vi "prueba.vi"() -> ()   [LabVIEW 2020]
uses:
  <vilib>/userDefined/High Color/IMAQdx.ctl
  <vilib>/vision/driver/NI_Vision_Acquisition_Software.lvlib
panel:
  in  "confirmar":bool
  in  "Session In":T1
  in  "stop":bool
  out "Image":T2(plugin-control)
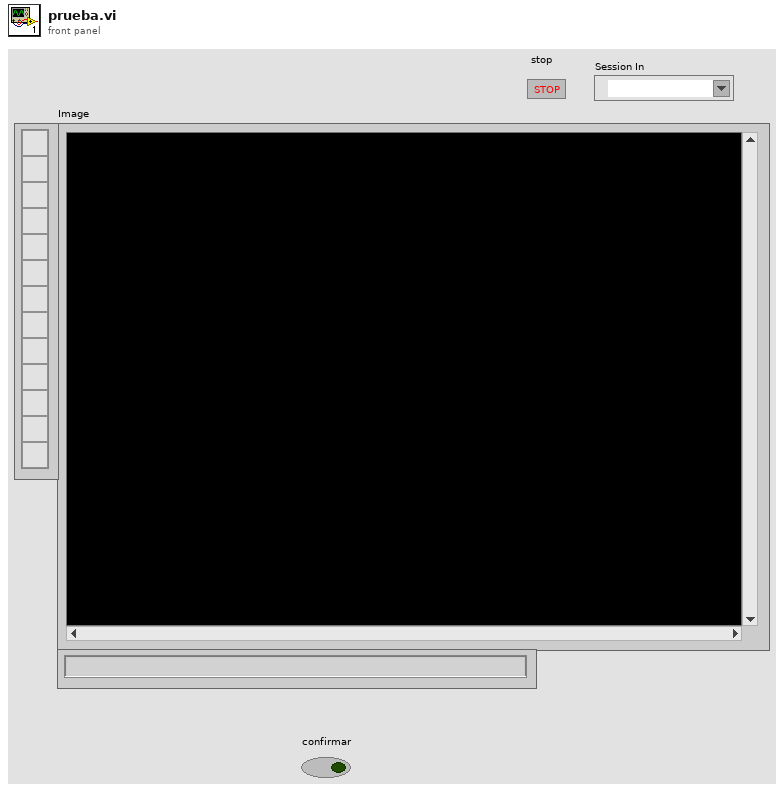
[diagram p1: front panel]
types:
  T1 = typedef "IMAQdx.ctl" = refnum<k21>
  T2 = typedef "IMAQ Image.ctl" = refnum<image>
  T3 = typedef "Image Type" = u32
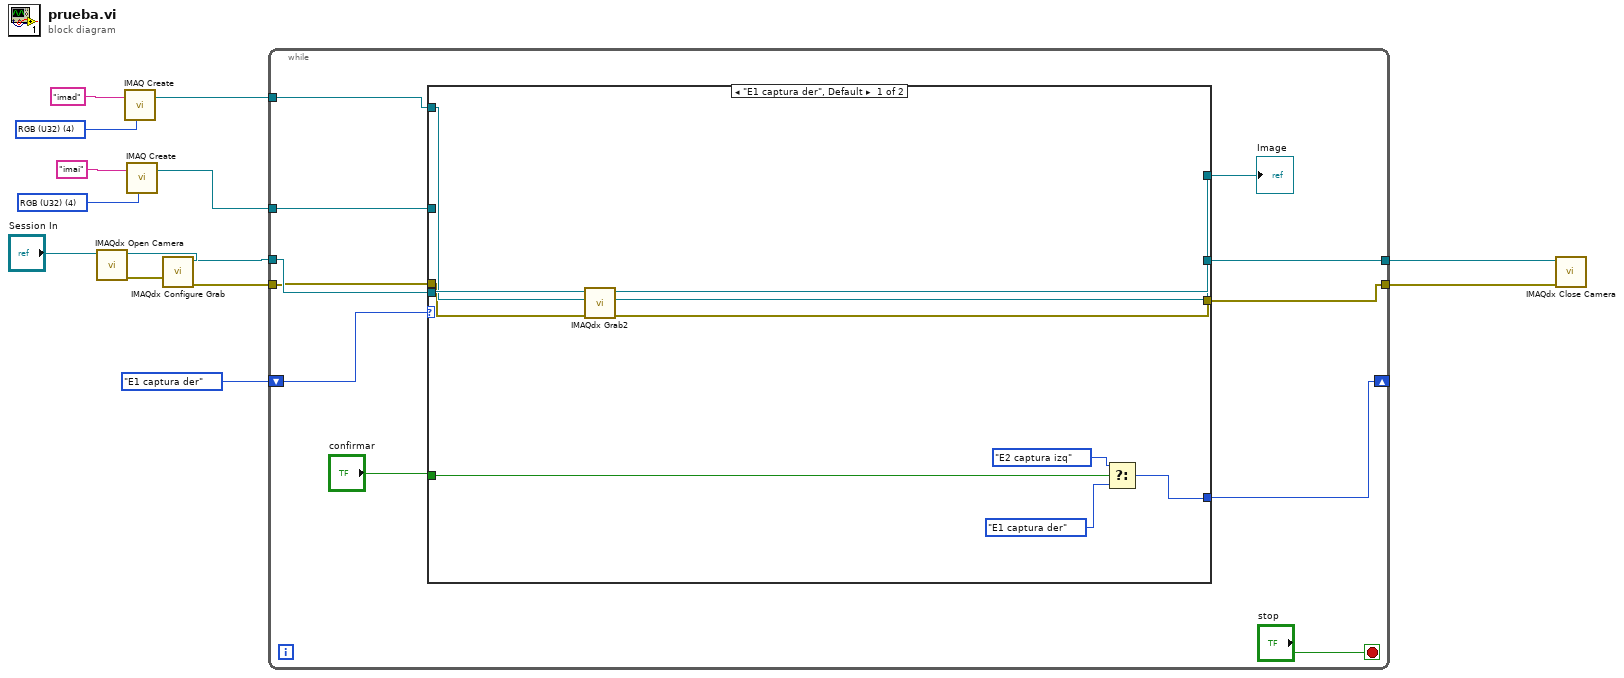
[diagram p0: block diagram]
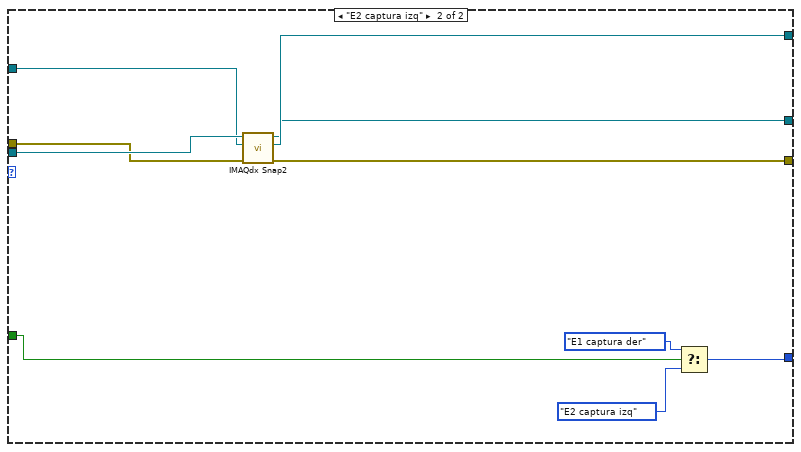
[diagram p2: hidden frame]
diagram:
  w7 = T3 4 items=["Grayscale (U8)", "Grayscale (I16)", "Grayscale (SGL)", "Complex (CSG)", "RGB (U32)", "HSL (U32)", "RGB (U64)", "Grayscale (U16)"] ("Image Type")
  w9 = T3 4 items=["Grayscale (U8)", "Grayscale (I16)", "Grayscale (SGL)", "Complex (CSG)", "RGB (U32)", "HSL (U32)", "RGB (U64)", "Grayscale (U16)"] ("Image Type")
  n1 = call <vilib>:"IMAQdx Open Camera.vi"("Session In"="Session In") -> ("error out"=w13:errorcluster, "Session Out"=w14:T1)  [unwired: 9 in]
  n2 = call "IMAQ Create"("Image Name"="imad", "Image Type"=w9) -> ("New Image"=w5:T2)  [unwired: 3 in, 1 out]
  n3 = call "IMAQ Create"("Image Name"="imai", "Image Type"=w7) -> ("New Image"=w6:T2)  [unwired: 3 in, 1 out]
  n4 = call <vilib>:"IMAQdx Configure Grab.vi"("error in"=w13, "Session In"=w14) -> ("error out"=w3:errorcluster, "Session Out"=w4:T1)  [unwired: 8 in]
  n5 = while {
    tunnel: w6 -> [w15]
    tunnel: w5 -> [w22]
    tunnel: w4 -> [w23]
    tunnel: w3 -> [w21]
    tunnel: [w20] -> w2
    tunnel: [w18] -> w1
    shift-right: [w17] -> _
    shift-left: enum16{"E1 captura der", "E2 captura izq"}."E1 captura der" -> [w25]
    stop <- "stop" stop-if-true
    n6 = case shown="\"E1 captura der\", Default" w25 {
      tunnel: w23 -> [w35 w45]
      tunnel: w22 -> [w34 _]
      tunnel: w21 -> [w33 w44]
      tunnel: [w31 w43] -> w20
      tunnel: [w30 w42] -> w19
      tunnel: [w32 w41] -> w18
      tunnel: [w29 w38] -> w17
      tunnel: "confirmar" -> [w26 w37]
      tunnel: w15 -> [_ w36]
      frame "E1 captura der", Default {
        n7 = call <vilib>:"IMAQdx Grab2.vi"("error in"=w33, "Image In"=w34, "Session In"=w35) -> ("error out"=w31:errorcluster, "Image Out"=w30:T2, "Session Out"=w32:T1)  [unwired: 5 in, 1 out]
        n8 = Select(t=enum16{"E1 captura der", "E2 captura izq"}."E2 captura izq", s=w26, f=enum16{"E1 captura der", "E2 captura izq"}."E1 captura der") -> (s? t:f=w29:enum16{"E1 captura der", "E2 captura izq"})
      }
      frame "E2 captura izq" {
        n9 = call <vilib>:"IMAQdx Snap2.vi"("error in"=w44, "Image In"=w36, "Session In"=w45) -> ("error out"=w43:errorcluster, "Image Out"=w42:T2, "Session Out"=w41:T1)  [unwired: 6 in]
        n10 = Select(t=enum16{"E1 captura der", "E2 captura izq"}."E1 captura der", s=w37, f=enum16{"E1 captura der", "E2 captura izq"}."E2 captura izq") -> (s? t:f=w38:enum16{"E1 captura der", "E2 captura izq"})
      }
    }
    "Image" <- w19
  }
  n11 = call <vilib>:"IMAQdx Close Camera.vi"("error in"=w2, "Session In"=w1) -> ()  [unwired: 9 in, 1 out]
